vi "Engine In - Sensor - Oil Level Switch.vi"(10 "Loop Freq [Hz]":sgl, 11 "Oil Level Switch [Ohm]":sgl) -> (3 "Oil Level Switch [OFF=OK]":bool)   [LabVIEW 2015, in "ECS-RT.lvlib"]
uses:
  ECS-RT.lvlib
  <vilib>/ptbypt/NI_PtbyPt.lvlib
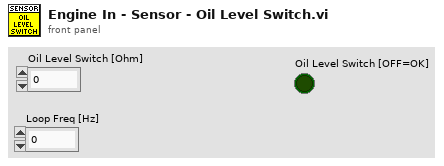
[diagram p1: front panel]
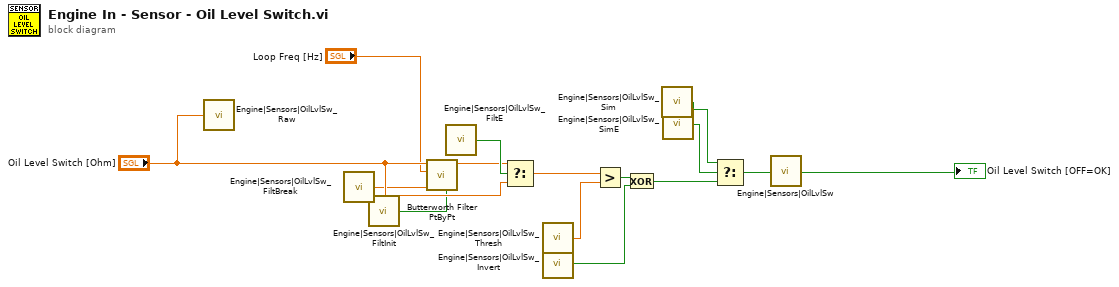
[diagram p0: block diagram]
diagram:
  n1 = call "Engine|Sensors|OilLvlSw_Raw"("Value"="Oil Level Switch [Ohm]") -> ()
  n2 = call "Engine|Sensors|OilLvlSw_FiltBreak"() -> ("Value"=w11:sgl)
  n3 = call "Engine|Sensors|OilLvlSw_FiltInit"() -> ("Value"=w9:bool)
  n4 = call <vilib>:"Butterworth Filter PtByPt.vi"("initialize"=w9, "low cutoff freq: fl"=w11, "sampling freq: fs"="Loop Freq [Hz]", "x"="Oil Level Switch [Ohm]") -> ("Filtered x"=w10:dbl)  [unwired: 5 in, 1 out]
  n5 = call "Engine|Sensors|OilLvlSw_FiltE"() -> ("Value"=w12:bool)
  n6 = Select(t=w10, s=w12, f="Oil Level Switch [Ohm]") -> (s? t:f=w5:dbl)
  n7 = call "Engine|Sensors|OilLvlSw_Thresh"() -> ("Value"=w6:sgl)
  n8 = call "Engine|Sensors|OilLvlSw_Invert"() -> ("Value"=w3:bool)
  n9 = Greater?(x=w5, y=w6) -> (0:w4:bool)
  n10 = Exclusive Or(1:w3, 2:w4) -> (0:w2:bool)
  n11 = call "Engine|Sensors|OilLvlSw_Sim"() -> ("Value"=w7:bool)
  n12 = call "Engine|Sensors|OilLvlSw_SimE"() -> ("Value"=w13:bool)
  n13 = Select(t=w7, s=w13, f=w2) -> (s? t:f=w1:bool)
  "Oil Level Switch [OFF=OK]" <- w1
  n14 = call "Engine|Sensors|OilLvlSw"("Value"=w1) -> ()
